vi "ConfigDisplayLastRowListBox.vi"(10 "Array":string[][](array[string]), 11 "reference":refnum<vi>) -> ()   [LabVIEW 2018, in "Config.lvlib"]
uses:
  Config.lvlib
  <vilib>/Utility/miscctls.llb/LVRowAndColumnTypeDef.ctl
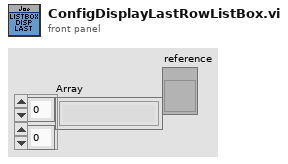
[diagram p1: front panel]
types:
  T1 = typedef "LVRowAndColumnTypeDef.ctl" = cluster{"Row":i32, "Column":i32}
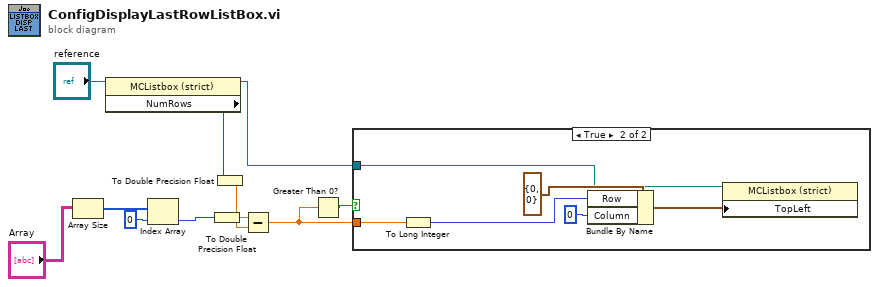
[diagram p0: block diagram]
diagram:
  n1 = Array Size(array="Array") -> (size(s)=w7:i32[])
  n2 = property on="Property Node" class="MCListbox (strict)"(reference="reference") -> (reference out=w11:refnum<vi>, "NumRows"=w8:u32)  [unwired: 1 in, 1 out]
  n3 = Index Array(array=w7, index=0) -> (element=w9:i32)
  n4 = To Double Precision Float(number=w9) -> (double precision float=w3:dbl)
  n5 = To Double Precision Float(number=w8) -> (double precision float=w4:dbl)
  n6 = Subtract(x=w3, y=w4) -> (x-y=w1:dbl)
  n7 = Greater Than 0?(x=w1) -> (x > 0?=w2:bool)
  n8 = case shown="True" w2 {
    tunnel: w1 -> [_ w14]
    tunnel: w11 -> [_ w13]
    frame False {
    }
    frame True {
      n9 = To Long Integer(number=w14) -> (32bit integer=w12:i32)
      n10 = Bundle By Name(cluster=T1 {"Row"=0, "Column"=0} ("Edit Position"), "Row"=w12, "Column"=0) -> (w16:T1)
      n11 = property on="Property Node" class="MCListbox (strict)"(reference=w13, "TopLeft"=w16) -> ()  [unwired: 1 in, 2 out]
    }
  }
